vi "Yield Error (async).vi"(4 "ArgumentsKw":string, 6 "Arguments":string, 7 "Options":string, 8 "Error in":errorcluster, 9 "Error URI":string, 10 "Invoation Request":refnum<class "Invocation Request ID.lvclass">, 11 "WAMP Client in":refnum<class "WAMP Client.lvclass">) -> (0 "Error out":errorcluster, 3 "WAMP Client out":refnum<class "WAMP Client.lvclass">)   [LabVIEW 2020, in "wamplv.lvlib" / "WAMP Client.lvclass"]
uses:
  WAMP Client.lvclass
  WAMP Client.lvclass/WAMP Client.ctl
  Private/TypeDef/Internal Message Type.ctl
  TypeDefs/WAMP error.ctl
  Private/TypeDefs/WAMP Message Codes.ctl
  wamplv.lvlib
  Private/TypeDef/Error Request.ctl
  Private/Invocation Request ID/Invocation Request ID.lvclass
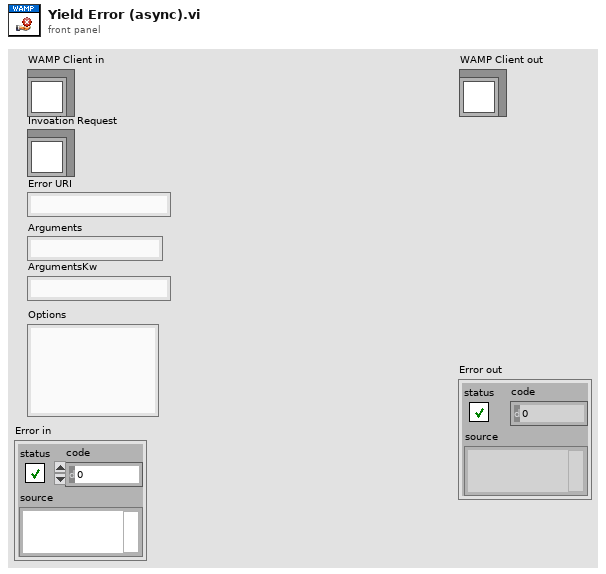
[diagram p1: front panel]
types:
  T1 = typedef "wamplv.lvlib/WAMP Client.lvclass/WAMP error.ctl" = cluster{"Details":string, "ArgumentKw Payload":string, "Error?":bool, "Error URI":string, "Arguments Payload":string}
  T2 = typedef "wamplv.lvlib/WAMP Client.lvclass/Error Request.ctl" = cluster{"WAMP Error":T1, "Message Type":T3, "Request ID":u64}
  T3 = typedef "wamplv.lvlib/WAMP Message Codes.ctl" = u16
  T4 = typedef "wamplv.lvlib/WAMP Client.lvclass/Internal Message Type.ctl" = enum16{"Subscribe", "Handle Subscribed", "Handle Event", "Unsubscribe", "Handle Unsubscribed", "Publish", "Handled Published", "Goodbye", "Handle Goodbye", "Call", "Handle Result", "Register", "Handle Registered", "Unregister", "Handle Unregistered", "Handle Invocation", "Yield", "Error"}
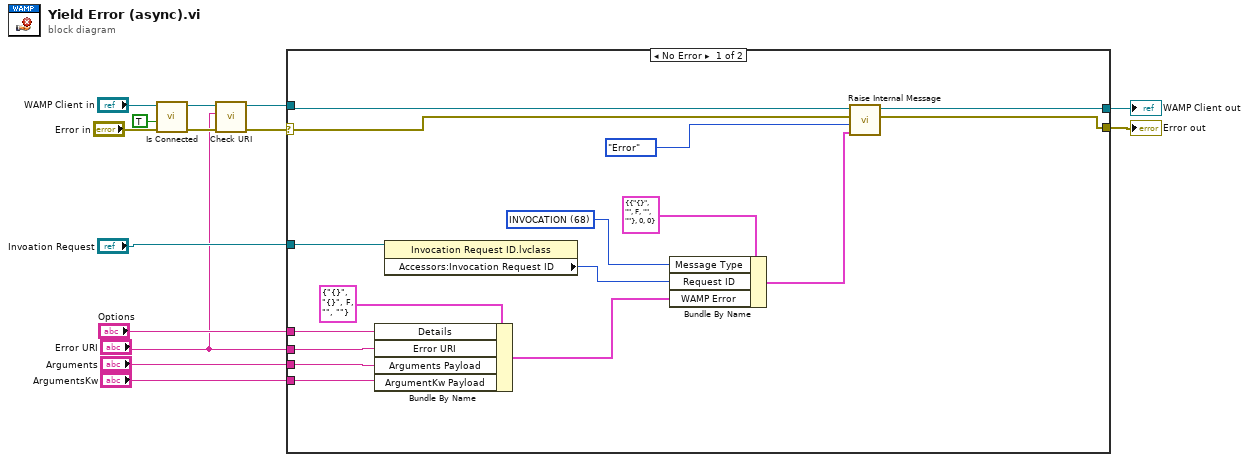
[diagram p0: block diagram]
diagram:
  n1 = call "Is Connected.vi"("error in"="Error in", "Raise error if not connected"=TRUE, "WAMP Client in"="WAMP Client in") -> ("error out"=w5:errorcluster, "WAMP Client out"=w3:refnum<class "WAMP Client.lvclass">)  [unwired: 6 in, 1 out]
  n2 = call "Check URI.vi"("error in (no error)"=w5, "URI"="Error URI", "WAMP Client in"=w3) -> ("error out"=w4:errorcluster, "WAMP Client out"=w2:refnum<class "WAMP Client.lvclass">)  [unwired: 5 in, 2 out]
  n3 = case shown="No Error" w4 {
    selector: w4 -> [w26 w32]
    tunnel: [w27 w32] -> w14
    tunnel: [w29 w31] -> w13
    tunnel: w2 -> [w30 w31]
    tunnel: "ArgumentsKw" -> [w21 _]
    tunnel: "Options" -> [w22 _]
    tunnel: "Error URI" -> [w20 _]
    tunnel: "Arguments" -> [w19 _]
    tunnel: "Invoation Request" -> [w16 _]
    frame No Error {
      w24 = T3 68 items=["HELLO"=1, "WELCOME"=2, "ABORT"=3, "GOODBYE"=6, "ERROR"=8, "PUBLISH"=16, "PUBLISHED"=17, "SUBSCRIBE"=32, "SUBSCRIBED"=33, "UNSUBSCRIBE"=34, "UNSUBSCRIBED"=35, "EVENT"=36, "CALL"=48, "RESULT"=59, "REGISTER"=64, "REGISTERED"=65, "UNREGISTER"=66, "UNREGISTERED"=67, "INVOCATION"=68, "YIELD"=70] ("Message Type")
      n4 = Bundle By Name(cluster=T1 {"Details"="{}", "ArgumentKw Payload"="{}", "Error?"=FALSE, "Error URI"="", "Arguments Payload"=""} ("WAMP Error"), "Details"=w22, "Error URI"=w20, "Arguments Payload"=w19, "ArgumentKw Payload"=w21) -> (w18:T1)
      n5 = property class="Invocation Request ID.lvclass"(reference=w16) -> ("Accessors:Invocation Request ID"=w15:u64)  [unwired: 1 in, 2 out]
      n6 = Bundle By Name(cluster=T2 {"WAMP Error"={"Details"="{}", "ArgumentKw Payload"="", "Error?"=FALSE, "Error URI"="", "Arguments Payload"=""}, "Message Type"=0, "Request ID"=0} ("Error Request"), "Message Type"=w24, "Request ID"=w15, "WAMP Error"=w18) -> (w17:T2)
      n7 = call "Raise Internal Message.vi"("Variant"=w17, "Internal Message Type"=Internal_Message_Type."Error", "error in (no error)"=w26, "WAMP Client in"=w30) -> ("error out"=w27:errorcluster, "WAMP Client out"=w29:refnum<class "WAMP Client.lvclass">)  [unwired: 6 in]
    }
    frame Error {
    }
  }
  "Error out" <- w14
  "WAMP Client out" <- w13
